vi "Read IoU.vi"(8 "error in (no error)":errorcluster, 11 "ONNX YOLO Class in":refnum<class "ONNX YOLO Class.lvclass">) -> (0 "error out":errorcluster, 2 "IoU":sgl, 3 "ONNX YOLO Class out":refnum<class "ONNX YOLO Class.lvclass">)   [LabVIEW 2017, in "ONNX YOLO Class Library.lvlib" / "ONNX YOLO Class.lvclass"]
uses:
  ONNX YOLO Class.lvclass
  ONNX YOLO Class.lvclass/ONNX YOLO Class.ctl
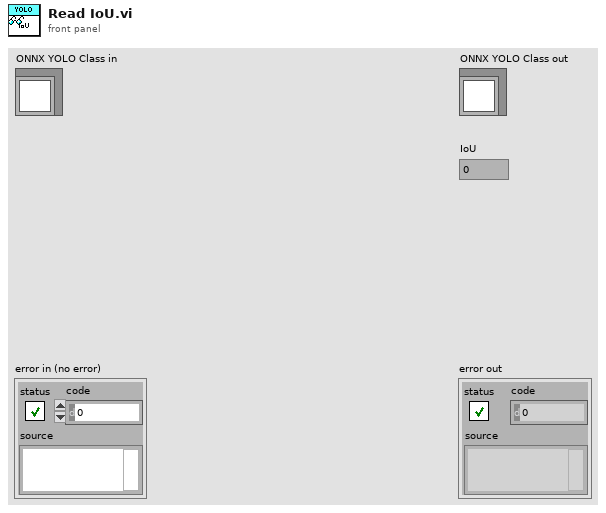
[diagram p1: front panel]
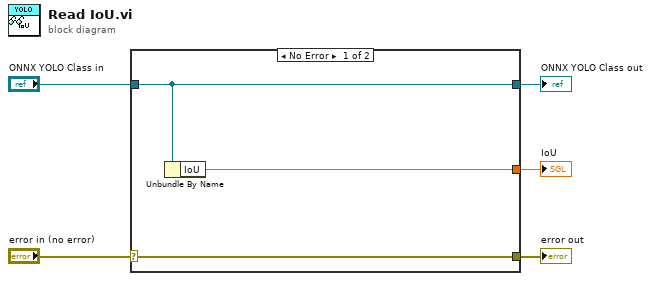
[diagram p0: block diagram]
diagram:
  n1 = case shown="No Error" "error in (no error)" {
    selector: "error in (no error)" -> [w8 w9]
    tunnel: [w8 w9] -> w4
    tunnel: [w7 w10] -> w2
    tunnel: "ONNX YOLO Class in" -> [w7 w10]
    tunnel: [w6 _] -> w1
    frame No Error {
      n2 = Unbundle By Name(w7) -> ("IoU"=w6:sgl)
    }
    frame Error {
    }
  }
  "error out" <- w4
  "ONNX YOLO Class out" <- w2
  "IoU" <- w1
